vi "Handle LogRec.vi"(8 "error in":errorcluster, 10 "LogRecord":refnum<class "LogRecord.lvclass">, 11 "NetworkHandler in":refnum<class "StreamLogHandle.lvclass">) -> (0 "error out":errorcluster, 3 "NetworkHandler out":refnum<class "StreamLogHandle.lvclass">)   [LabVIEW 2024]
doc: "Handles the incoming ``LogRecord`` object. If the level of the record is greater or equal to the level of the handler, then the record is written to the file. \n\n____\nHAMPEL SOFTWARE ENGINEERING v2.2.2 (2025-01-16 15:41)"
uses:
  StreamLogHandle.lvclass/StreamLogHandle.ctl
  <vilib>/Hampel Software Engineering/HSE Logger/LogRecord/LogRecord.lvclass
  <vilib>/Utility/error.llb/whitespace.ctl
  <vilib>/Hampel Software Engineering/HSE Logger/Formatter/Formatter.lvclass
  Stream/INetworkWriter/INetworkWriter.lvclass
  StreamLogHandle.lvclass
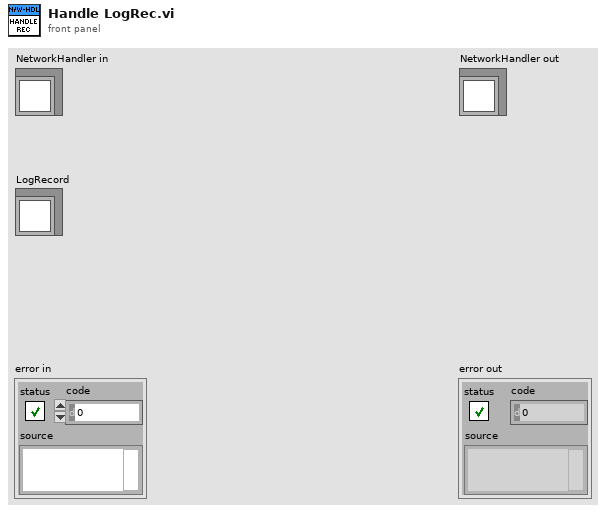
[diagram p1: front panel]
types:
  T1 = typedef "hse-logger.lvlib/LogLevel.ctl" = enum16{"DEBUG", "INFO", "WARNING", "ERROR", "CRITICAL"}
  T2 = typedef "whitespace.ctl" = u16
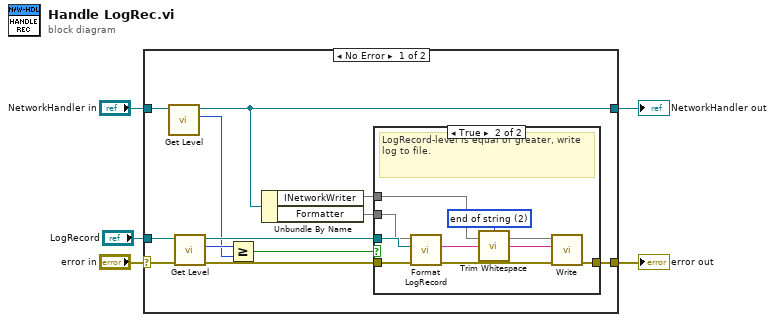
[diagram p0: block diagram]
diagram:
  n1 = case shown="No Error" "error in" {
    selector: "error in" -> [w17 w29]
    tunnel: [w7 w29] -> w4
    tunnel: [w9 w28] -> w2
    tunnel: "NetworkHandler in" -> [w14 w28]
    tunnel: "LogRecord" -> [w16 _]
    frame No Error {
      n2 = call-dynamic <vilib>:"Get Level.vi"("Handler in"=w14) -> ("Level"=w12:T1, "Handler out"=w9:refnum<class "NetworkHandler.lvclass">)  [unwired: 8 in, 1 out]
      n3 = call <vilib>:"Get Level.vi"("error in"=w17, "LogRecord in"=w16) -> ("error out"=w8:errorcluster, "Level"=w13:T1, "LogRecord out"=w15:refnum<class "LogRecord.lvclass">)  [unwired: 7 in]
      n4 = Greater Or Equal?(x=w13, y=w12) -> (x >= y?=w11:bool)
      n5 = Unbundle By Name(w9) -> ("INetworkWriter"=w10, "Formatter"=w6)
      n6 = case shown="True" w11 {
        tunnel: w15 -> [_ w26]
        tunnel: w8 -> [w18 w27]
        tunnel: [w18 w21] -> w7
        tunnel: w10 -> [_ w24]
        tunnel: w6 -> [_ w25]
        frame False {
          # "Do not write to file."
        }
        frame True {
          w19 = T2 2 items=["both", "start of string", "end of string"] ("location (both)")
          # "LogRecord-level is equal or greater, write log to file."
          n7 = call-dynamic "Format LogRecord.vi"("error in"=w27, "LogRecord"=w26, "Formatter in"=w25) -> ("error out"=w22:errorcluster, "LogLine"=w23:string)  [unwired: 7 in]
          n8 = call <vilib>:"Trim Whitespace.vi"("string"=w23, "location (both)"=w19) -> ("trimmed string"=w20:string)
          n9 = call-dynamic "Write.vi"("error in (no error)"=w22, "Message"=w20, "INetworkWriter in"=w24) -> ("error out"=w21:errorcluster)  [unwired: 7 in, 1 out]
        }
      }
    }
    frame Error {
    }
  }
  "error out" <- w4
  "NetworkHandler out" <- w2
